vi "Send Command.vi"(7 "Config offset":u64 format="%x", 8 "error in (no error)":errorcluster, 9 "Command payload":u64 format="%x", 10 "Command number":T1, 11 "RP Communicator in":refnum<class "RP Communicator.lvclass">) -> (0 "error out":errorcluster, 3 "RP Communicator out":refnum<class "RP Communicator.lvclass">)   [LabVIEW 2018, in "RP Communicator.lvclass"]
uses:
  RP Communicator.lvclass
  RP Command.ctl
  RP Communicator.lvclass/RP Communicator.ctl
  Read Timeout.vi
  RP Write Command TCP.vi
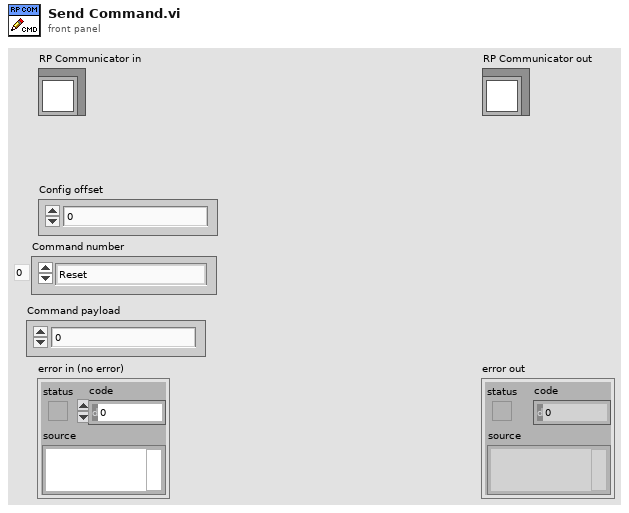
[diagram p1: front panel]
types:
  T1 = typedef "RP Command.ctl" = enum16{"Reset", "Read IDN", "Stop server", "Get status", "Get temperature", "Connect client", "Arm", "Software trigger", "Get whole buffer", "Get chunk", "System call", "Get config", "Set config", "Recieve data", "Recieve Calibartion", "Transmit data"}
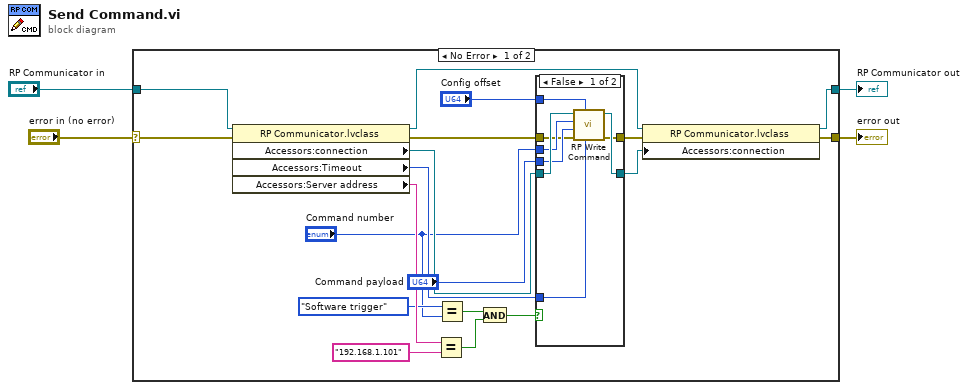
[diagram p0: block diagram]
diagram:
  n1 = case shown="No Error" "error in (no error)" {
    selector: "error in (no error)" -> [w16 w35]
    tunnel: [w13 w35] -> w3
    tunnel: [w18 w34] -> w1
    tunnel: "RP Communicator in" -> [w20 w34]
    frame No Error {
      n2 = property class="RP Communicator.lvclass"(reference=w20, error in=w16) -> (reference out=w19:refnum<class "RP Communicator.lvclass">, error out=w15:errorcluster, "Accessors:connection"=w23:refnum<k5>, "Accessors:Timeout"=w12:i32, "Accessors:Server address"=w10:string)
      n3 = Equal?(x=w10, y="192.168.1.101") -> (x = y?=w9:bool)
      n4 = Equal?(x=RP_Command."Software trigger" ("Command number"), y="Command number") -> (x = y?=w5:bool)
      n5 = And(x=w5, y=w9) -> (x .and. y?=w6:bool)
      n6 = case shown="False" w6 {
        tunnel: w23 -> [w31 w32]
        tunnel: "Config offset" -> [w30 _]
        tunnel: "Command number" -> [w29 _]
        tunnel: "Command payload" -> [w28 _]
        tunnel: [w27 w32] -> w17
        tunnel: w15 -> [w26 w33]
        tunnel: [w25 w33] -> w14
        tunnel: w12 -> [w24 _]
        frame False {
          n7 = call-poly "RP Write Command.vi"("timeout ms (25000)"=w24, "Config offset"=w30, "Error In"=w26, "Command payload"=w28, "Command number"=w29, "connection ID"=w31) -> ("Error Out"=w25:errorcluster, "connection ID out"=w27:refnum<k5>)  [unwired: 3 in, 1 out]
        }
        frame True {
        }
      }
      n8 = property class="RP Communicator.lvclass"(reference=w19, error in=w14, "Accessors:connection"=w17) -> (reference out=w18:refnum<class "RP Communicator.lvclass">, error out=w13:errorcluster)
    }
    frame Error {
    }
  }
  "error out" <- w3
  "RP Communicator out" <- w1
